vi "setupActuator.vi"(8 "error in (no error)":errorcluster, 10 "Model in":refnum<class "Model.lvclass">, 11 "Bootloader in":refnum<class "Bootloader.lvclass">) -> (0 "error out":errorcluster, 2 "Model out":refnum<class "Model.lvclass">, 3 "Bootloader out":refnum<class "Bootloader.lvclass">)   [LabVIEW 2015, in "Bootloader.lvclass"]
uses:
  Bootloader.lvclass
  Model/Model.lvclass
  Actuator/PressureServoActuator/PressureServoActuator.lvclass
  ActuatorCylinder/ILCControlledActuatorCylinder/ILCControlledActuatorCylinder.lvclass
  ILCDACFactory/ILCDACFactory/ILCDACFactory.lvclass
  Typedefs/Pressure Servo Settings.ctl
  Typedefs/DAC Settings.ctl
  Calculators/VoltageToILCDACRaw/VoltageToILCDACRaw.lvclass
  Calculators/VoltageToILCDACRaw/VoltageToILCDACRaw.lvclass/VoltageToILCDACRaw.ctl
  Actuator/PressureServoActuator/PressureServoActuator.lvclass/PressureServoActuator.ctl
  ActuatorCylinder/ILCControlledActuatorCylinder/ILCControlledActuatorCylinder.lvclass/ILCControlledActuatorCylinder.ctl
  Model/Model.lvclass/Model.ctl
  ConfigurationTestParameters/ConfigurationTestParameters.lvclass
  Typedefs/FAMTTypedefs.lvlib
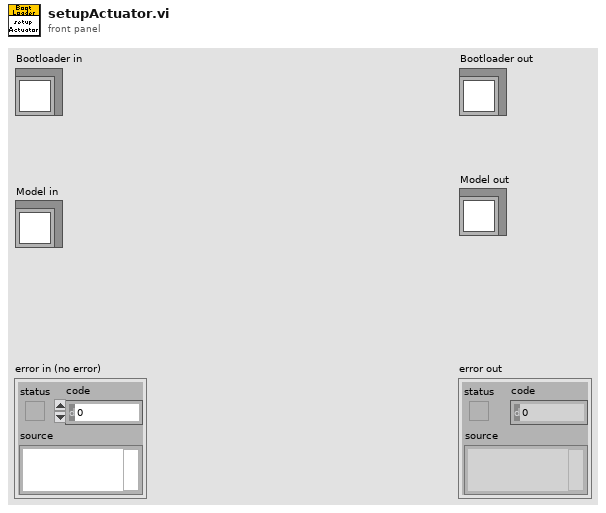
[diagram p1: front panel]
types:
  T1 = typedef "FAMTTypedefs.lvlib/DAC Settings.ctl" = cluster{"Voltage Reference":dbl[unit], "Min Counts":i32, "Max Counts":i32}
  T2 = typedef "FAMTTypedefs.lvlib/Pressure Servo Settings.ctl" = cluster{"Center Point":dbl[unit], "Area":dbl, "PA to PSI":dbl, "Servo 1 DAC Channel":u8, "Servo 2 DAC Channel":u8}
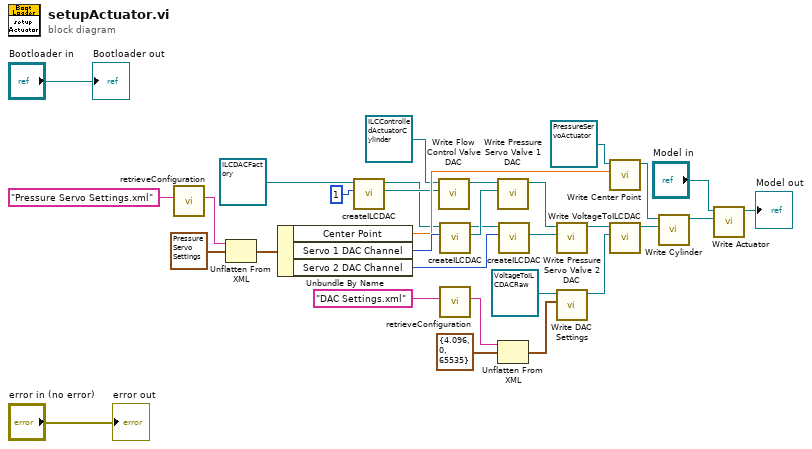
[diagram p0: block diagram]
diagram:
  n1 = call "retrieveConfiguration.vi"("configName"="Pressure Servo Settings.xml") -> ("xmlConfig"=w17:string)  [unwired: 8 in, 2 out]
  n2 = Unflatten From XML(xml string=w17, type=T2 {"Center Point"=413685.4733709468, "Area"=0.004536, "PA to PSI"=0.000145038, "Servo 1 DAC Channel"=1, "Servo 2 DAC Channel"=2} ("Pressure Servo Settings")) -> (value=w19:T2)  [unwired: 1 in, 1 out]
  n3 = Unbundle By Name(w19) -> ("Center Point"=w20:dbl[unit], "Servo 1 DAC Channel"=w21:u8, "Servo 2 DAC Channel"=w22:u8)
  n4 = call-dynamic "createILCDAC.vi"("Channel"=u8 1, "ILCDACFactory in"=refnum<class "ILCDACFactory.lvclass"> refnum ("ILCDACFactory.lvclass")) -> ("ILCDAC"=w10:refnum<class "IILCDAC.lvclass">, "ILCDACFactory out"=w8:refnum<class "ILCDACFactory.lvclass">)  [unwired: 7 in, 1 out]
  n5 = call "Write Flow Control Valve DAC.vi"("IILCDAC"=w10, "ILCControlledActuatorCylinder in"=refnum<class "ILCControlledActuatorCylinder.lvclass"> refnum ("ILCControlledActuatorCylinder.lvclass")) -> ("ILCControlledActuatorCylinder out"=w5:refnum<class "ILCControlledActuatorCylinder.lvclass">)  [unwired: 9 in]
  n6 = call-dynamic "createILCDAC.vi"("Channel"=w21, "ILCDACFactory in"=w8) -> ("ILCDAC"=w11:refnum<class "IILCDAC.lvclass">, "ILCDACFactory out"=w9:refnum<class "ILCDACFactory.lvclass">)  [unwired: 7 in, 1 out]
  n7 = call "retrieveConfiguration.vi"("configName"="DAC Settings.xml") -> ("xmlConfig"=w24:string)  [unwired: 8 in, 2 out]
  n8 = call "Write Pressure Servo Valve 1 DAC.vi"("IILCDAC"=w11, "ILCControlledActuatorCylinder in"=w5) -> ("ILCControlledActuatorCylinder out"=w4:refnum<class "ILCControlledActuatorCylinder.lvclass">)  [unwired: 9 in]
  n9 = Unflatten From XML(xml string=w24, type=T1 {"Voltage Reference"=4.096, "Min Counts"=0, "Max Counts"=65535} ("DAC Settings")) -> (value=w29:T1)  [unwired: 1 in, 1 out]
  n10 = call-dynamic "createILCDAC.vi"("Channel"=w22, "ILCDACFactory in"=w9) -> ("ILCDAC"=w12:refnum<class "IILCDAC.lvclass">)  [unwired: 7 in, 2 out]
  n11 = call "Write Pressure Servo Valve 2 DAC.vi"("IILCDAC"=w12, "ILCControlledActuatorCylinder in"=w4) -> ("ILCControlledActuatorCylinder out"=w26:refnum<class "ILCControlledActuatorCylinder.lvclass">)  [unwired: 9 in]
  n12 = call "Write DAC Settings.vi"("DAC Settings"=w29, "VoltageToILCDACRaw in"=refnum<class "VoltageToILCDACRaw.lvclass"> refnum ("VoltageToILCDACRaw.lvclass")) -> ("VoltageToILCDACRaw out"=w30:refnum<class "VoltageToILCDACRaw.lvclass">)  [unwired: 9 in]
  n13 = call "Write Center Point.vi"("Center Point"=w20, "PressureServoActuator in"=refnum<class "PressureServoActuator.lvclass"> refnum ("PressureServoCylinderActuator.lvclass")) -> ("PressureServoActuator out"=w15:refnum<class "PressureServoActuator.lvclass">)  [unwired: 9 in]
  n14 = call "Write VoltageToILCDAC.vi"("VoltageToILCDAC"=w30, "ILCControlledActuatorCylinder in"=w26) -> ("ILCControlledActuatorCylinder out"=w27:refnum<class "ILCControlledActuatorCylinder.lvclass">)  [unwired: 9 in]
  n15 = call "Write Cylinder.vi"("ActuatorCylinder"=w27, "PressureServoActuator in"=w15) -> ("PressureServoActuator out"=w3:refnum<class "PressureServoActuator.lvclass">)  [unwired: 9 in]
  n16 = call "Write Actuator.vi"("IActuator.lvclass"=w3, "Model in"="Model in") -> ("Model out"=→"Model out":refnum<class "Model.lvclass">)  [unwired: 9 in]
  "error out" <- "error in (no error)"
  "Bootloader out" <- "Bootloader in"
